vi "Escape String for Python.vi"(10 "String":string) -> (2 "Escaped Python String":string)   [LabVIEW 2020, in "jki_python_data_tools.lvlib"]
uses:
  jki_python_data_tools.lvlib
panel:
  # "Copyright © 2003-2009 JKI. All rights reserved.\n\nAuthor: Jim Kring [jim.kring@jameskring.com]\n\nThis library is provided \"AS IS\" ,WITHOUT WARRANTIES OR \nCONDITIONS OF ANY KIND, either express or implied.\n\nJames Kring, Inc. -- http://www.jameskring.com"
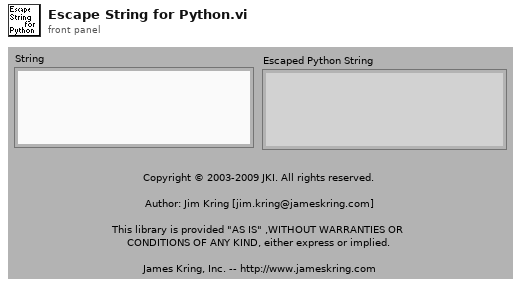
[diagram p1: front panel]
types:
  T1 = cluster{"Char ('\\' Codes Display)":string, "Escape Code (Normal Display)":string}[]
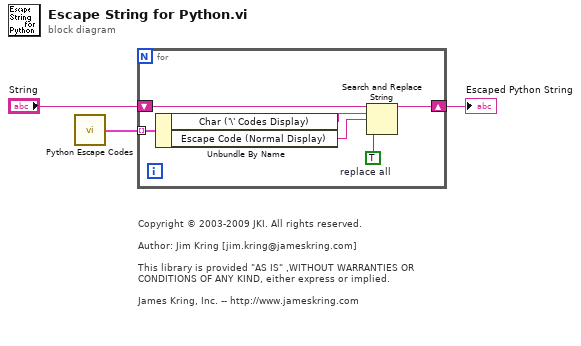
[diagram p0: block diagram]
diagram:
  # "Copyright © 2003-2009 JKI. All rights reserved.\n\nAuthor: Jim Kring [jim.kring@jameskring.com]\n\nThis library is provided \"AS IS\" ,WITHOUT WARRANTIES OR \nCONDITIONS OF ANY KIND, either express or implied.\n\nJames Kring, Inc. -- http://www.jameskring.com"
  n1 = call "Python Escape Codes.vi"() -> ("Python Escape Codes"=w3:T1)
  n2 = for {
    shift-right: [w8] -> w1
    shift-left: "String" -> [w9]
    tunnel: w3 -> [w6] mode=indexing
    w7 = TRUE  # replace all
    n3 = Unbundle By Name(w6) -> ("Char ('\\' Codes Display)"=w5:string, "Escape Code (Normal Display)"=w4:string)
    n4 = Search and Replace String(replace all?=w7, input string=w9, search string=w5, replace string=w4) -> (result string=w8:string)  [unwired: 4 in, 3 out]
  }
  "Escaped Python String" <- w1
